vi "data_swap.vi"(10 "data in":dbl[](array[numeric]), 11 "data bus in":T1) -> (2 "data out":dbl[](array[numeric]), 3 "data bus out":T1)   [LabVIEW 2024, in "IPE Optimization Tester.lvlib"]
uses:
  IPE Optimization Tester.lvlib
  data_bus--cluster.ctl
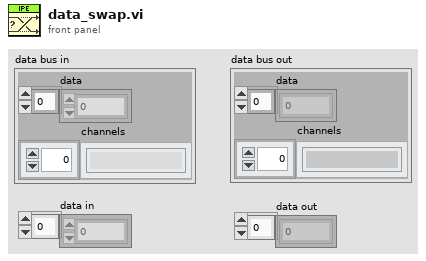
[diagram p1: front panel]
types:
  T1 = typedef "IPE Optimization Tester.lvlib/data_bus--cluster.ctl" = cluster{"data":dbl[], "channels":string[]}
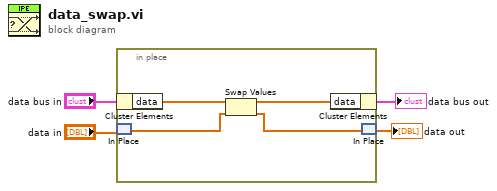
[diagram p0: block diagram]
diagram:
  n1 = in-place {
    n2 = in-place-cluster #1("data bus in") -> ("data"=w8:dbl[])
    n3 = in-place-match #2("data in") -> (w6:dbl[])
    n4 = Swap Values(12:w8, 14:w6) -> (1:w7:dbl[], 3:w5:dbl[])  [unwired: 1 in]
    n5 = in-place-cluster #1("data"=w7) -> (→"data bus out":T1)
    n6 = in-place-match #2(w5) -> (→"data out":dbl[])
  }
